vi "TWG_Query.vi"(0 "System no.":i32=1 min=1 max=4 step=1, 5 "error in":errorcluster) -> (14 "Number of wave generators":i32, 19 "error out":errorcluster)   [LabVIEW 2020]
doc: "Returns the number of available wave generators.\n\nC-413: Number of wave generators = 2\n\nC-887: Number of wave generators = No. of connected axes. \n\nC-891: Number of wave generators = 1\n\nE-517, E-518: Number of wave generators = 3\n\nE-709: Number of wave generators = 1\n\nE-710: Number of wave generators = 2\n\nE-712: Number of wave generators = No. of connected axes\n\nE-725, E-727: Number of wave generators = No. of connected axes\n\nE-753: Number of wave generators = 1\n\nE-754: Number of wave generators = 1\n\nE-761: Number of wave generators = 4"
panel:
  # "Returns the number of available wave generators."
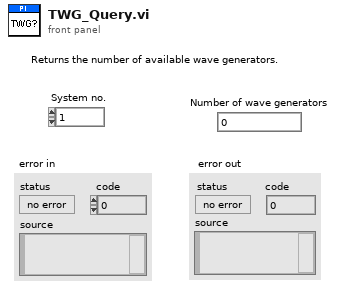
[diagram p1: front panel]
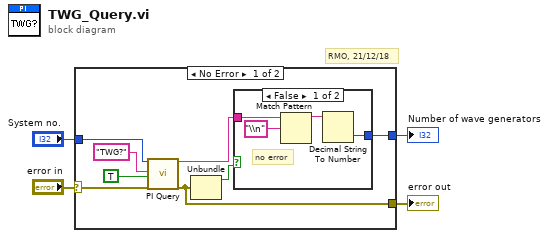
[diagram p0: block diagram]
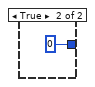
[diagram p2: hidden frame]
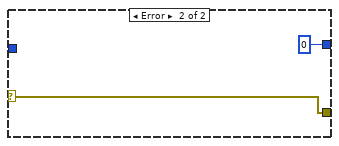
[diagram p3: hidden frame]
diagram:
  # "RMO, 21/12/18"
  n1 = case shown="No Error" "error in" {
    selector: "error in" -> [w5 w19]
    tunnel: [w11 0] -> w4
    tunnel: "System no." -> [w9 _]
    tunnel: [w7 w19] -> w2
    frame No Error {
      n2 = call "PI Query.vi"("System no."=w9, "String to send"="TWG?", "Attach termination char.?"=TRUE ("Attach Linefeed?"), "error in"=w5) -> ("String read"=w6:string, "error out"=w7:errorcluster)  [unwired: 3 in, 11 out]
      n3 = Unbundle(w7) -> ("status"=w12:bool)  [unwired: 2 out]
      n4 = case shown="False" w12 {
        tunnel: w6 -> [w15 _]
        tunnel: [w16 0] -> w11
        frame False {
          # "no error"
          n5 = Match Pattern(string=w15, regular expression="\\n") -> (before substring=w13:string)  [unwired: 4 out]
          n6 = Decimal String To Number(string=w13) -> (number=w16:i32)  [unwired: 3 out]
        }
        frame True {
        }
      }
    }
    frame Error {
    }
  }
  "error out" <- w2
  "Number of wave generators" <- w4
